vi "programa13.vi"() -> ()   [LabVIEW 2011]
panel:
  in  "Stop":bool
  out "Foco":bool
  in  "On/Off":bool
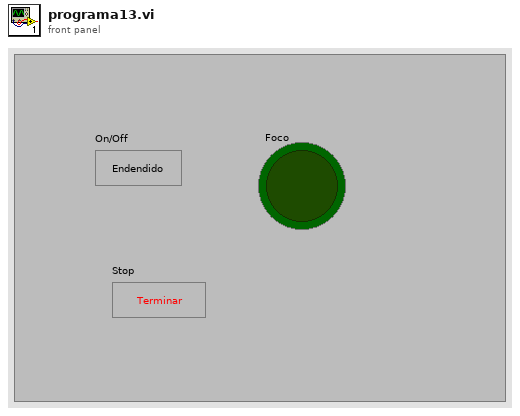
[diagram p1: front panel]
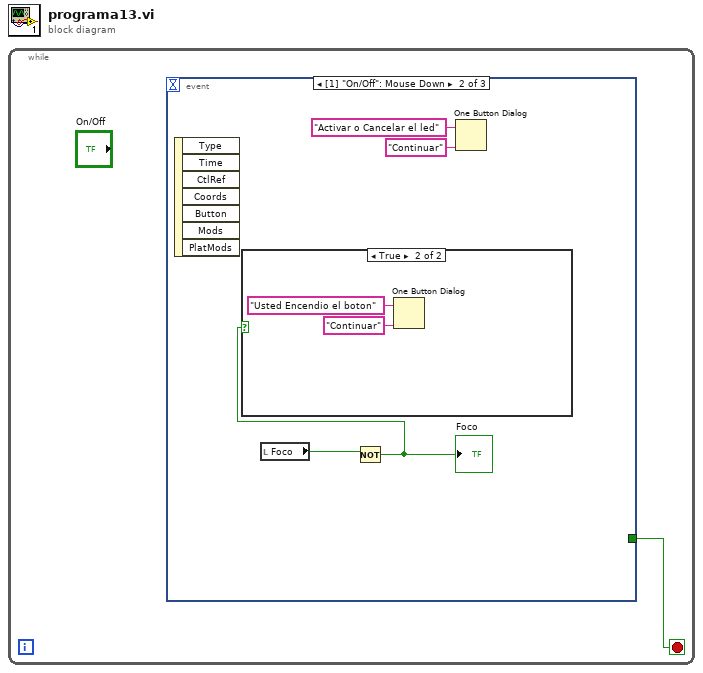
[diagram p0: block diagram]
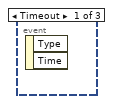
[diagram p2: hidden frame]
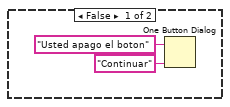
[diagram p3: hidden frame]
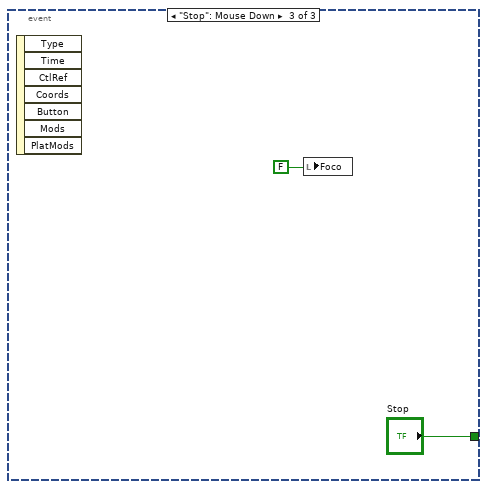
[diagram p4: hidden frame]
diagram:
  n1 = while {
    stop <- w1 stop-if-true
    n2 = event shown="[1] \"On/Off\": Mouse Down" {
      selector: _ -> [_ _ _]
      dyn-events: _ -> [_ _ _]
      timeout: _ -> [_ _ _]
      tunnel: [_ _ "Stop"] -> w1
      event Timeout {
        n3 = event-data() -> ()  [unwired: 1 in, 2 out]
      }
      event "On/Off": Mouse Down {
        n4 = event-data() -> ()  [unwired: 1 in, 7 out]
        n5 = local read "Foco"() -> (w5:bool)
        n6 = Not(x=w5) -> (.not. x?=w2:bool)
        "Foco" <- w2
        n7 = case shown="True" w2 {
          frame False {
            n8 = One Button Dialog(message="Usted apago el boton", button name ("OK")="Continuar") -> ()  [unwired: 1 out]
          }
          frame True {
            n9 = One Button Dialog(message="Usted Encendio el boton", button name ("OK")="Continuar") -> ()  [unwired: 1 out]
          }
        }
        n10 = One Button Dialog(message="Activar o Cancelar el led", button name ("OK")="Continuar") -> ()  [unwired: 1 out]
      }
      event "Stop": Mouse Down {
        n11 = event-data() -> ()  [unwired: 1 in, 7 out]
        n12 = local write "Foco"(FALSE) -> ()
      }
    }
  }
